vi "Load Controller Plugins.vi"(11 "Shuwdown Event":refnum<user-event>) -> (3 "Controller Plugins":refnum<class "Controller Interface.lvclass">[](array[class]))   [LabVIEW 2019]
uses:
  Controller Interface/Controller Interface.lvlibp/Controller Interface Class/Controller Interface.lvclass
  <vilib>/Utility/LVLibp/NI_PackedLibraryUtility.lvlib
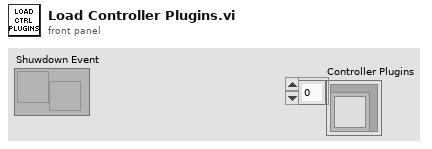
[diagram p1: front panel]
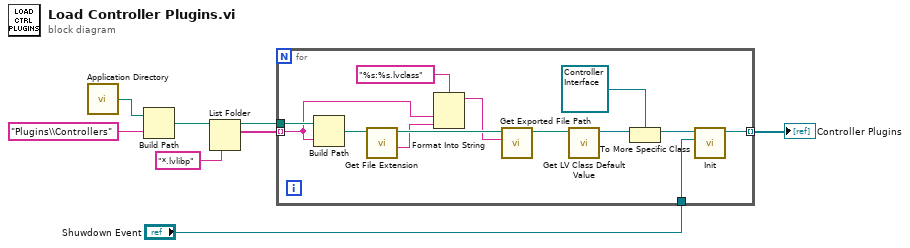
[diagram p0: block diagram]
diagram:
  n1 = call <vilib>:"Application Directory.vi"() -> ("Application Directory"=w8:path)
  n2 = Build Path(base path=w8, name or relative path="Plugins\\Controllers") -> (appended path=w6:path)
  n3 = List Folder(path=w6, pattern="*.lvlibp") -> (path out=w4:path, filenames=w5:string[])  [unwired: 2 in, 2 out]
  n4 = for {
    tunnel: w5 -> [w16] mode=indexing
    tunnel: w4 -> [w21]
    tunnel: [w10] -> w3 mode=indexing
    tunnel: "Shuwdown Event" -> [w9]
    n5 = Build Path(base path=w21, name or relative path=w16) -> (appended path=w20:path)
    n6 = call <vilib>:"Get File Extension.vi"("file"=w20) -> ("filename without extension"=w15:string, "dup file"=w19:path)  [unwired: 6 in, 3 out]
    n7 = Format Into String(format string="%s:%s.lvclass", w16, w15) -> (resulting string=w17:string)  [unwired: 2 in, 1 out]
    n8 = call <vilib>:"Get Exported File Path.vi"("qualified name"=w17, "packed library path"=w19) -> ("path"=w14:path)  [unwired: 8 in, 1 out]
    n9 = call <vilib>:"Get LV Class Default Value.vi"("class path"=w14) -> ("object"=w13:refnum<class>)  [unwired: 9 in, 1 out]
    n10 = To More Specific Class(target class=refnum<class "Controller Interface.lvclass"> refnum ("Controller Interface.lvlibp:Controller Interface.lvclass"), reference=w13) -> (specific class reference=w11:refnum<class "Controller Interface.lvclass">)  [unwired: 1 in, 1 out]
    n11 = call-dynamic "Init.vi"("Shuwdown Event"=w9, "Controller Interface in"=w11) -> ("Controller Interface out"=w10:refnum<class "Controller Interface.lvclass">)  [unwired: 8 in, 1 out]
  }
  "Controller Plugins" <- w3
